vi "Read configuration.vi"(8 "error in":errorcluster, 11 "Calculated Tags editor node in":refnum<class "Calculated Tags editor node.lvclass">) -> (0 "error out":errorcluster, 2 "configuration":refnum<class "NISE_CEF_serializable configuration.lvclass">, 3 "Calculated Tags editor node out":refnum<class "Calculated Tags editor node.lvclass">)   [LabVIEW 2014, in "Calculated Tags editor node.lvclass"]
uses:
  Calculated Tags editor node.lvclass
  <vilib>/NI/Configuration Framework/serializable configuration/NISE_CEF_serializable configuration.lvclass
  Calculated Tags editor node.lvclass/Calculated Tags editor node.ctl
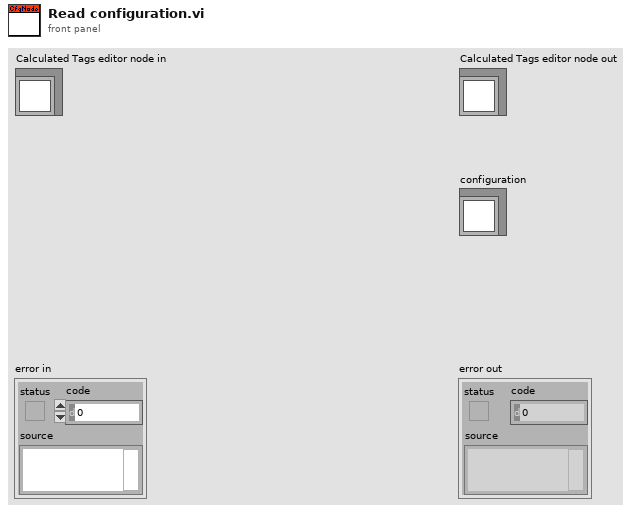
[diagram p1: front panel]
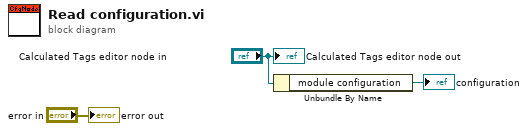
[diagram p0: block diagram]
diagram:
  n1 = Unbundle By Name("Calculated Tags editor node in") -> ("module configuration"=→"configuration":refnum<class "Calculated Tags configuration.lvclass">)
  "error out" <- "error in"
  "Calculated Tags editor node out" <- "Calculated Tags editor node in"
